vi "Read Configuration OO.vi"() -> ()   [LabVIEW 2014, in "LVOOP Introduction.lvlib"]
doc: "Read object oriented configuration data from ini-file using the configuration class.\n\nLizenziert unter EUPL V. 1.1"
uses:
  LVOOP Introduction.lvlib
  Configuration/Classes/Configuration/Configuration.lvclass
  Configuration/Classes/Ini-File/Ini-File.lvclass
panel:
  out "Sections":T1(array[cluster])
  out "Configuration out":refnum<class "Configuration.lvclass">
  in  "Configuration File Path":path
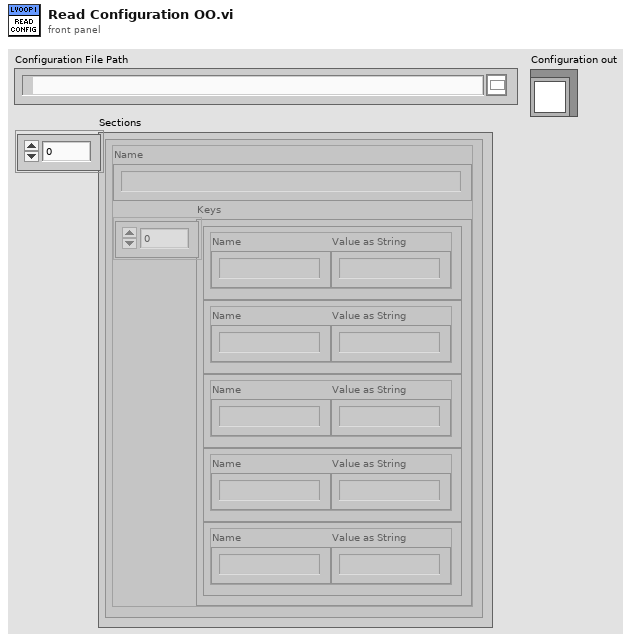
[diagram p1: front panel]
types:
  T1 = cluster{"Name":string, "Keys":cluster{"Name":string, "Value as String":string}[]}[]
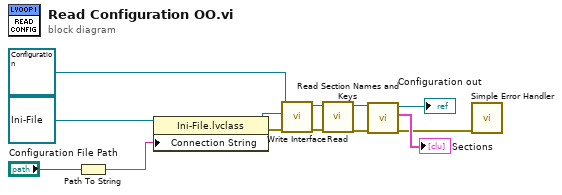
[diagram p0: block diagram]
diagram:
  n1 = Path To String(path="Configuration File Path") -> (string=w5:string)
  n2 = property class="Ini-File.lvclass"(reference=refnum<class "Ini-File.lvclass"> refnum ("Configuration.lvlib:Ini-File.lvclass"), "Connection String"=w5) -> (reference out=w1:refnum<class "Ini-File.lvclass">, error out=w12:errorcluster)  [unwired: 1 in]
  n3 = call "Write Interface.vi"("error in (no error)"=w12, "Interface"=w1, "Configuration in"=refnum<class "Configuration.lvclass"> refnum) -> ("error out"=w11:errorcluster, "Configuration out"=w10:refnum<class "Configuration.lvclass">)  [unwired: 7 in]
  n4 = call "Read.vi"("error in (no error)"=w11, "Configuration"=w10) -> ("error out"=w2:errorcluster, "Configuration out"=w3:refnum<class "Configuration.lvclass">)  [unwired: 8 in]
  n5 = call "Read Section Names and Keys.vi"("error in (no error)"=w2, "Configuration in"=w3) -> ("error out"=w6:errorcluster, "Sections"=→"Sections":T1, "Configuration out"=→"Configuration out":refnum<class "Configuration.lvclass">)  [unwired: 7 in]
  n6 = call <vilib>:"Simple Error Handler.vi"("error in (no error)"=w6) -> ()  [unwired: 4 in, 5 out]
